vi "Time BenchmarkGen.vi"() -> ()   [LabVIEW 2019]
panel:
  out "size":i32=1000000000
  out "x-y":u32
  out "Delta(ms) 2":u32
  out "Delta(ms)":u32
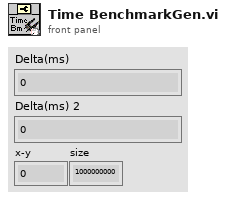
[diagram p1: front panel]
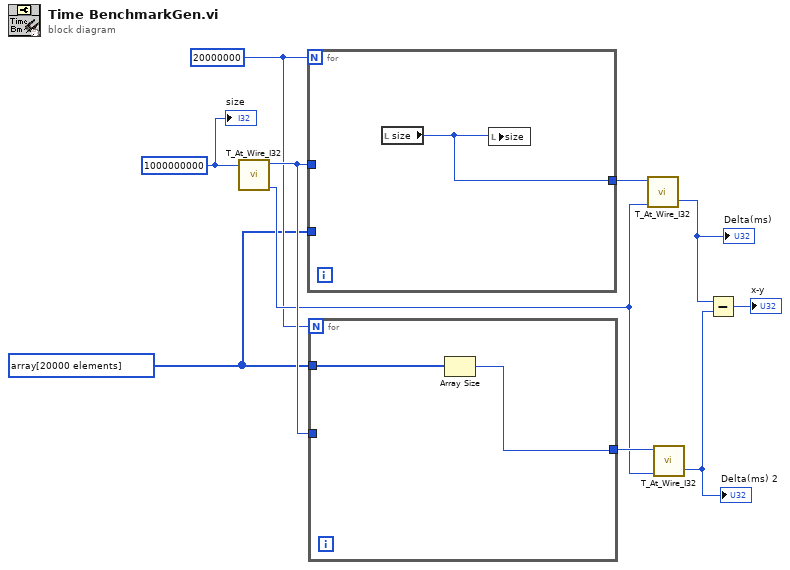
[diagram p0: block diagram]
diagram:
  w2 = i32[] array[20000 elements]
  w6 = 20000000
  w10 = 1000000000 ("y")
  n1 = call <userlib>:"T_At_Wire_I32.vi"("I32"=w10) -> ("Clock(ms)"=w7:u32, "I32 Out"=w9:i32)  [unwired: 8 in, 1 out]
  n2 = for {
    N: w6 -> [_]
    tunnel: w9 -> [_]
    tunnel: w2 -> [_]
    tunnel: [w11] -> w1
    n3 = local read "size"() -> (w11:i32)
    n4 = local write "size"(w11) -> ()
  }
  n5 = for {
    N: w6 -> [_]
    tunnel: w9 -> [_]
    tunnel: [w12] -> w8
    tunnel: w2 -> [w13]
    n6 = Array Size(array=w13) -> (size(s)=w12:i32)
  }
  n7 = call <userlib>:"T_At_Wire_I32.vi"("InitClock(ms)"=w7, "I32"=w1) -> ("Delta(ms)"=w5:u32)  [unwired: 7 in, 2 out]
  "Delta(ms)" <- w5
  n8 = call <userlib>:"T_At_Wire_I32.vi"("InitClock(ms)"=w7, "I32"=w8) -> ("Delta(ms)"=w4:u32)  [unwired: 7 in, 2 out]
  "Delta(ms) 2" <- w4
  n9 = Subtract(x=w5, y=w4) -> (x-y=→"x-y":u32)
  "size" <- w10
